vi "frameratetest.vi"() -> ()   [LabVIEW 2019]
panel:
  out "Software FPS":dbl
  out "Camera FPS":dbl
  out "Image":u16[][](graph)
  out "Camera Serial":string
  out "Camera Version":string
  out "Camera Model":string
  out "SMD":dbl
  in  "Scan Mode":dbl min=1.0 max=2.0 step=1.0
  in  "Exposure":dbl min=0.0010036691729323308 max=10.000004210526317 step=1e-08
  out "EXP":dbl
  out "SVW":i32
  out "SHW":i32
  out "SVO":i32
  out "SHO":i32
  in  "V Width":i32 min=2 max=528 step=2
  in  "V Offset":i32 min=0 max=992 step=2
  in  "H Width":i32 min=2 max=1024 step=2
  in  "H Offset":i32 min=0 max=992 step=2
  in  "Binning":u16(ring)=1 items=["1x1"=1, "2x2"=2, "4x4"=4]
  out "Elapsed Time":u32
  out "Total Frames":i32
  in  "Display":bool=TRUE
  out "error out":errorcluster
  in  "stop":bool
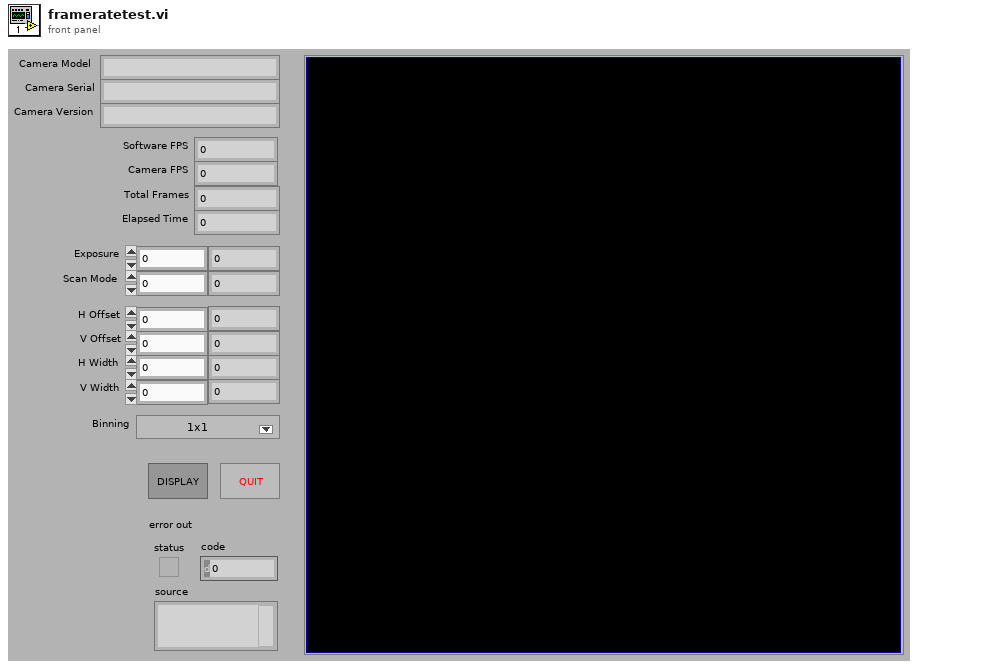
[diagram p1: front panel]
types:
  T1 = cluster{"Model":string, "Camera ID":string, "Firmware":string}
  T2 = typedef "LVMinMaxIncTypeDef.ctl" = cluster{"Minimum":dbl, "Maximum":dbl, "Increment":dbl}
  T3 = cluster{"H Offset":cluster{"Value":i32, "Limits":T2}, "V Offset":cluster{"Value":i32, "Limits":T2}, "H Size":cluster{"Value":i32, "Limits":T2}, "V Size":cluster{"Value":i32, "Limits":T2}}
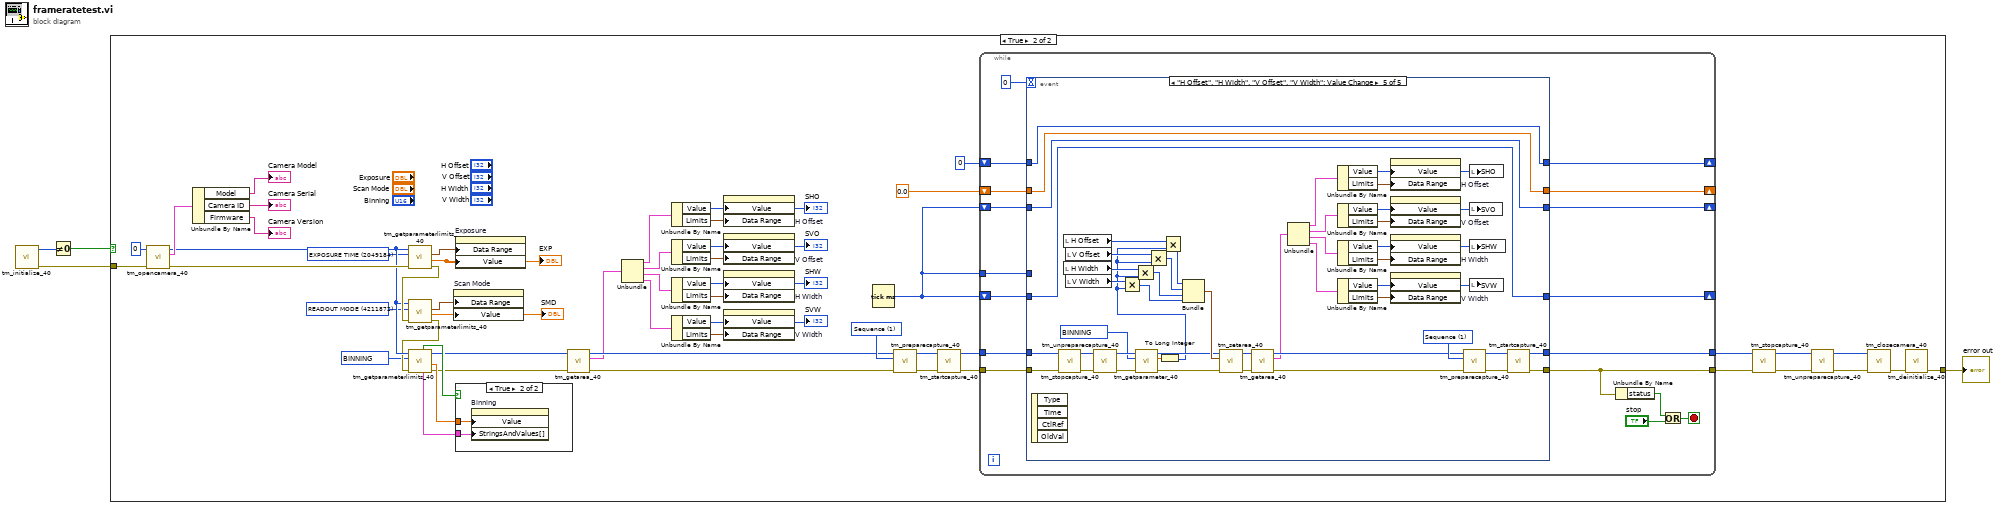
[diagram p0: block diagram]
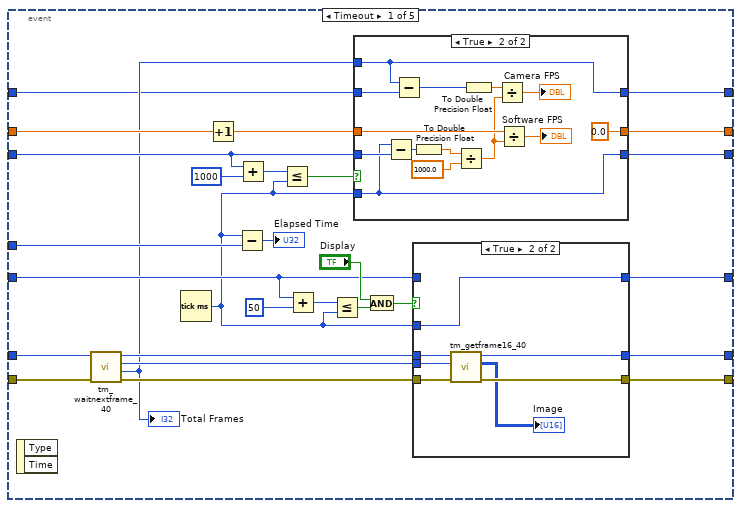
[diagram p4: hidden frame]
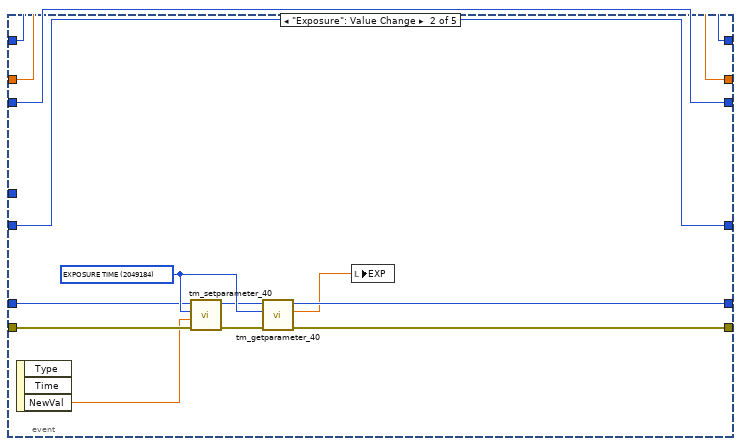
[diagram p7: hidden frame]
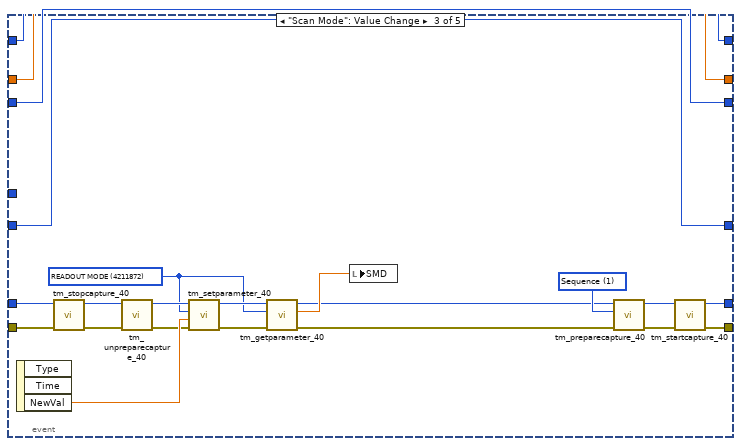
[diagram p8: hidden frame]
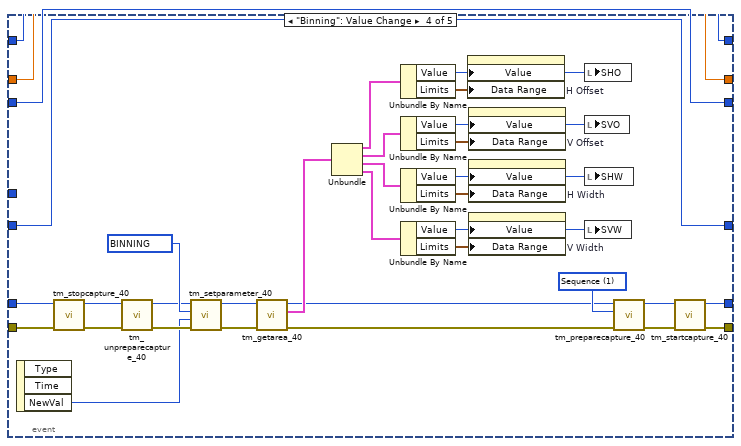
[diagram p9: hidden frame]
diagram:
  n1 = call <userlib>:"tm_initialize_40.vi"() -> ("error out"=w2:errorcluster, "Number Of Cameras"=w1:u32)  [unwired: 8 in, 2 out]
  n2 = Not Equal To 0?(x=w1) -> (x != 0?=w4:bool)
  n3 = case shown="True" w4 {
    tunnel: [w5 w55] -> w3
    tunnel: w2 -> [w5 w58]
    frame False {
    }
    frame True {
      w27 = u32 2049184 items=["BINNING"=4215968, "BITS PER CHANNEL"=4342976, "ACTIVE VIEW INDEX"=4343136, "CCD MODE"=4212384, "SENSOR MODE"=4212128, "READOUT MODE"=4211872, "EXPOSURE TIME"=2049184, "CONTRAST GAIN"=3163312, "CONTRAST OFFSET"=3163328, "LIGHT MODE"=2114720, "SENSITIVITY"=2114992, "WHITE BALANCE"=3163568, "PHOTON IMAGING MODE"=2115200, "HIGH DYNAMIC RANGE MODE"=3163360, "TRIGGER SOURCE"=1066144, "TRIGGER ACTIVE"=1066160, "TRIGGER MODE"=1066400, "TRIGGER POLARITY"=1066416, "TRIGGER GLOBAL EXPOSURE"=2049680, "FIRST TRIGGER BEHAVIOR"=2049696, "TRIGGER TIMES"=1066448, "OUTPUT TRIGGER POLARITY"=1852592, "OUTPUT TRIGGER DELAY"=1852624, "OUTPUT TRIGGER PERIOD"=1852640, "TEMPERATURE"=2115232, "TEMPERATURE TARGET"=2115264, "SENSOR COOLER FAN"=2115296, "MECHANICAL SHUTTER"=2115488, "BACK FOCUS POSITION"=8422304, "FRAMEBUNDLE MODE"=4346784, "FRAMEBUNDLE NUMBER"=4346800, "LINEBUNDLE HEIGHT"=4212192, "TRIGGER CONNECTOR"=1066432, "IMAGE PIXEL TYPE"=4343296, "OUTPUT TRIGGER KIND"=1852656, "READOUT DIRECTION"=4211904, "CHANNEL SYNC"=1852352] ("Parameter")
      w28 = u32 4211872 items=["BINNING"=4215968, "BITS PER CHANNEL"=4342976, "ACTIVE VIEW INDEX"=4343136, "CCD MODE"=4212384, "SENSOR MODE"=4212128, "READOUT MODE"=4211872, "EXPOSURE TIME"=2049184, "CONTRAST GAIN"=3163312, "CONTRAST OFFSET"=3163328, "LIGHT MODE"=2114720, "SENSITIVITY"=2114992, "WHITE BALANCE"=3163568, "PHOTON IMAGING MODE"=2115200, "HIGH DYNAMIC RANGE MODE"=3163360, "TRIGGER SOURCE"=1066144, "TRIGGER ACTIVE"=1066160, "TRIGGER MODE"=1066400, "TRIGGER POLARITY"=1066416, "TRIGGER GLOBAL EXPOSURE"=2049680, "FIRST TRIGGER BEHAVIOR"=2049696, "TRIGGER TIMES"=1066448, "OUTPUT TRIGGER POLARITY"=1852592, "OUTPUT TRIGGER DELAY"=1852624, "OUTPUT TRIGGER PERIOD"=1852640, "TEMPERATURE"=2115232, "TEMPERATURE TARGET"=2115264, "SENSOR COOLER FAN"=2115296, "MECHANICAL SHUTTER"=2115488, "BACK FOCUS POSITION"=8422304, "FRAMEBUNDLE MODE"=4346784, "FRAMEBUNDLE NUMBER"=4346800, "LINEBUNDLE HEIGHT"=4212192, "TRIGGER CONNECTOR"=1066432, "IMAGE PIXEL TYPE"=4343296, "OUTPUT TRIGGER KIND"=1852656, "READOUT DIRECTION"=4211904, "CHANNEL SYNC"=1852352] ("Parameter")
      w29 = u32 4215968 items=["BINNING"=4215968, "BITS PER CHANNEL"=4342976, "ACTIVE VIEW INDEX"=4343136, "CCD MODE"=4212384, "SENSOR MODE"=4212128, "READOUT MODE"=4211872, "EXPOSURE TIME"=2049184, "CONTRAST GAIN"=3163312, "CONTRAST OFFSET"=3163328, "LIGHT MODE"=2114720, "SENSITIVITY"=2114992, "WHITE BALANCE"=3163568, "PHOTON IMAGING MODE"=2115200, "HIGH DYNAMIC RANGE MODE"=3163360, "TRIGGER SOURCE"=1066144, "TRIGGER ACTIVE"=1066160, "TRIGGER MODE"=1066400, "TRIGGER POLARITY"=1066416, "TRIGGER GLOBAL EXPOSURE"=2049680, "FIRST TRIGGER BEHAVIOR"=2049696, "TRIGGER TIMES"=1066448, "OUTPUT TRIGGER POLARITY"=1852592, "OUTPUT TRIGGER DELAY"=1852624, "OUTPUT TRIGGER PERIOD"=1852640, "TEMPERATURE"=2115232, "TEMPERATURE TARGET"=2115264, "SENSOR COOLER FAN"=2115296, "MECHANICAL SHUTTER"=2115488, "BACK FOCUS POSITION"=8422304, "FRAMEBUNDLE MODE"=4346784, "FRAMEBUNDLE NUMBER"=4346800, "LINEBUNDLE HEIGHT"=4212192, "TRIGGER CONNECTOR"=1066432, "IMAGE PIXEL TYPE"=4343296, "OUTPUT TRIGGER KIND"=1852656, "READOUT DIRECTION"=4211904, "CHANNEL SYNC"=1852352] ("Parameter")
      w53 = 1 items=["Snap", "Sequence"] ("Capture mode")
      n4 = call <userlib>:"tm_opencamera_40.vi"("error in (no error)"=w58, "Camera Index"=u32 0) -> ("error out"=w36:errorcluster, "Camera Details"=w40:T1, "Handle out"=w34:u32)  [unwired: 7 in]
      n5 = Unbundle By Name(w40) -> ("Model"=→"Camera Model":string, "Camera ID"=→"Camera Serial":string, "Firmware"=→"Camera Version":string)
      n6 = call <userlib>:"tm_getparameterlimits_40.vi"("error in (no error)"=w36, "Parameter"=w27, "Handle in"=w34) -> ("error out"=w35:errorcluster, "default"=w19:dbl, "Range"=w20:cluster{"min":dbl, "max":dbl, "step":dbl})  [unwired: 2 in, 4 out]
      "EXP" <- w19
      n7 = call <userlib>:"tm_getparameterlimits_40.vi"("error in (no error)"=w35, "Parameter"=w28, "Handle in"=w34) -> ("error out"=w33:errorcluster, "default"=w21:dbl, "Range"=w22:cluster{"min":dbl, "max":dbl, "step":dbl})  [unwired: 2 in, 4 out]
      "SMD" <- w21
      n8 = call <userlib>:"tm_getparameterlimits_40.vi"("error in (no error)"=w33, "Parameter"=w29, "Handle in"=w34) -> ("error out"=w26:errorcluster, "default"=w31:dbl, "Handle out"=w25:u32, "Value Names"=w30:cluster{"Name":string, "Value":dbl}[], "Writable"=w32:bool)  [unwired: 2 in, 2 out]
      n9 = property on="Scan Mode" class="DigNum (strict)"("Data Range"=w22, "Value"=w21) -> ()  [unwired: 2 in, 2 out]
      n10 = property on="Exposure" class="DigNum (strict)"("Data Range"=w20, "Value"=w19) -> ()  [unwired: 2 in, 2 out]
      n11 = case shown="True" w32 {
        tunnel: w30 -> [_ w60]
        tunnel: w31 -> [_ w59]
        frame False {
        }
        frame True {
          n12 = property on="Binning" class="Ring (strict)"("Value"=w59, "StringsAndValues[]"=w60) -> ()  [unwired: 2 in, 2 out]
        }
      }
      n13 = call <userlib>:"tm_getarea_40.vi"("error in (no error)"=w26, "Handle in"=w25) -> ("error out"=w24:errorcluster, "Sub Region"=w14:T3, "Handle out"=w23:u32)  [unwired: 7 in]
      n14 = Unbundle(w14) -> ("H Offset"=w18:cluster{"Value":i32, "Limits":T2}, "V Offset"=w17:cluster{"Value":i32, "Limits":T2}, "H Size"=w16:cluster{"Value":i32, "Limits":T2}, "V Size"=w15:cluster{"Value":i32, "Limits":T2})
      n15 = Unbundle By Name(w18) -> ("Value"=w13:i32, "Limits"=w12:T2)
      "SHO" <- w13
      n16 = Unbundle By Name(w17) -> ("Value"=w7:i32, "Limits"=w6:T2)
      "SVO" <- w7
      n17 = Unbundle By Name(w16) -> ("Value"=w9:i32, "Limits"=w8:T2)
      "SHW" <- w9
      n18 = Unbundle By Name(w15) -> ("Value"=w11:i32, "Limits"=w10:T2)
      "SVW" <- w11
      n19 = property on="H Offset" class="DigNum (strict)"("Value"=w13, "Data Range"=w12) -> ()  [unwired: 2 in, 2 out]
      n20 = property on="V Offset" class="DigNum (strict)"("Value"=w7, "Data Range"=w6) -> ()  [unwired: 2 in, 2 out]
      n21 = property on="H Width" class="DigNum (strict)"("Value"=w9, "Data Range"=w8) -> ()  [unwired: 2 in, 2 out]
      n22 = property on="V Width" class="DigNum (strict)"("Value"=w11, "Data Range"=w10) -> ()  [unwired: 2 in, 2 out]
      n23 = Tick Count (ms)() -> (millisecond timer value=w48:u32)
      n24 = call <userlib>:"tm_preparecapture_40.vi"("error in (no error)"=w24, "Capture mode"=w53, "Handle in"=w23) -> ("error out"=w51:errorcluster, "Handle out"=w52:u32)  [unwired: 5 in, 2 out]
      n25 = call <userlib>:"tm_startcapture_40.vi"("error in (no error)"=w51, "Handle in"=w52) -> ("error out"=w50:errorcluster, "Handle out"=w49:u32)  [unwired: 8 in]
      n26 = while {
        tunnel: w50 -> [w67]
        tunnel: [w65] -> w47
        tunnel: [w64] -> w46
        shift-right: [w73] -> _
        shift-left: w48 -> [w71]
        shift-right: [w74] -> _
        shift-left: 0.0 -> [w72]
        shift-right: [w66] -> _
        shift-left: w48 -> [w69]
        tunnel: w49 -> [w68]
        tunnel: w48 -> [w70]
        shift-right: [w61] -> _
        shift-left: 0 -> [w62]
        stop <- w75 stop-if-true
        n27 = event shown="[4] \"H Offset\", \"H Width\", \"V Offset\", \"V Width\": Value Change" {
          selector: _ -> [_ _ _ _ _]
          dyn-events: _ -> [_ _ _ _ _]
          timeout: 0 -> [_ _ _ _ _]
          tunnel: [w82 w143 w165 w194 w240] -> w74
          tunnel: [w81 w144 w166 w195 w241] -> w73
          tunnel: w72 -> [w91 w143 w165 w194 w240]
          tunnel: w71 -> [w84 w144 w166 w195 w241]
          tunnel: w70 -> [w87 _ _ _ _]
          tunnel: w69 -> [w92 w145 w167 w201 w247]
          tunnel: w68 -> [w94 w138 w162 w193 w238]
          tunnel: w67 -> [w93 w140 w161 w192 w237]
          tunnel: [w90 w145 w167 w201 w247] -> w66
          tunnel: [w89 w135 w156 w196 w242] -> w65
          tunnel: [w88 w133 w157 w197 w243] -> w64
          tunnel: w62 -> [w79 w142 w155 w189 w234]
          tunnel: [w78 w142 w155 w189 w234] -> w61
          event Timeout {
            n28 = event-data() -> ()  [unwired: 1 in, 2 out]
            n29 = call <userlib>:"tm_waitnextframe_40.vi"("error in (no error)"=w93, "Handle in"=w94) -> ("error out"=w98:errorcluster, "Frame Count"=w80:i32, "Frame Index"=w97:i32, "Handle out"=w99:u32)  [unwired: 6 in]
            "Total Frames" <- w80
            n30 = Tick Count (ms)() -> (millisecond timer value=w86:u32)
            n31 = Increment(x=w91) -> (x+1=w83:dbl)
            n32 = Subtract(x=w86, y=w87) -> (x-y=→"Elapsed Time":u32)
            n33 = Add(x=w84, y=u32 1000) -> (x+y=w105:u32)
            n34 = Less Or Equal?(x=w105, y=w86) -> (x <= y?=w85:bool)
            n35 = Add(x=w92, y=u32 50) -> (x+y=w103:u32)
            n36 = Less Or Equal?(x=w103, y=w86) -> (x <= y?=w101:bool)
            n37 = case shown="True" w85 {
              tunnel: w84 -> [w108 w117]
              tunnel: [w108 w114] -> w81
              tunnel: w83 -> [w107 w120]
              tunnel: w86 -> [_ w114]
              tunnel: [w107 0.0] -> w82
              tunnel: w80 -> [_ w109]
              tunnel: w79 -> [w106 w112]
              tunnel: [w106 w109] -> w78
              frame False {
              }
              frame True {
                n38 = Subtract(x=w114, y=w117) -> (x-y=w116:u32)
                n39 = Subtract(x=w109, y=w112) -> (x-y=w110:i32)
                n40 = To Double Precision Float(number=w116) -> (double precision float=w122:dbl)
                n41 = Divide(x=w122, y=1000.0) -> (x/y=w113:dbl)
                n42 = To Double Precision Float(number=w110) -> (double precision float=w111:dbl)
                n43 = Divide(x=w111, y=w113) -> (x/y=→"Camera FPS":dbl)
                n44 = Divide(x=w120, y=w113) -> (x/y=→"Software FPS":dbl)
              }
            }
            n45 = And(x="Display", y=w101) -> (x .and. y?=w96:bool)
            n46 = case shown="True" w96 {
              tunnel: w92 -> [w125 _]
              tunnel: w86 -> [_ w132]
              tunnel: [w125 w132] -> w90
              tunnel: w99 -> [w124 w131]
              tunnel: w98 -> [w123 w130]
              tunnel: [w124 w129] -> w89
              tunnel: [w123 w128] -> w88
              tunnel: w97 -> [_ w126]
              frame False {
              }
              frame True {
                n47 = call <userlib>:"tm_getframe16_40.vi"("error in (no error)"=w130, "Frame Index"=w126, "Handle in"=w131) -> ("error out"=w128:errorcluster, "Data"=→"Image":u16[][], "Handle out"=w129:u32)  [unwired: 5 in, 1 out]
              }
            }
          }
          event "Exposure": Value Change {
            w141 = u32 2049184 items=["SENSOR MODE"=4212128, "CCD MODE"=4212384, "READOUT MODE"=4211872, "ACTIVE VIEW INDEX"=4343136, "BITS PER CHANNEL"=4342976, "IMAGE PIXEL TYPE"=4343296, "BINNING"=4215968, "EXPOSURE TIME"=2049184, "CONTRAST GAIN"=3163312, "CONTRAST OFFSET"=3163328, "LIGHT MODE"=2114720, "SENSITIVITY"=2114992, "PHOTON IMAGING MODE"=2115200, "HIGH DYNAMIC RANGE MODE"=3163360, "WHITE BALANCE"=3163568, "TEMPERATURE"=2115232, "TEMPERATURE TARGET"=2115264, "SENSOR COOLER FAN"=2115296, "LINEBUNDLE HEIGHT"=4212192, "MECHANICAL SHUTTER"=2115488, "BACK FOCUS POSITION"=8422304, "TRIGGER CONNECTOR"=1066432, "TRIGGER SOURCE"=1066144, "OUTPUT TRIGGER SOURCE"=1852576, "TRIGGER GLOBAL EXPOSURE"=2049680, "FIRST TRIGGER BEHAVIOR"=2049696, "CHANNEL SYNC"=1852352, "READOUT DIRECTION"=4211904, "PRE HSYNC COUNT"=1852704] ("Parameter")
            n48 = event-data() -> ("NewVal"=w139:dbl)  [unwired: 1 in, 2 out]
            n49 = call <userlib>:"tm_setparameter_40.vi"("error in (no error)"=w140, "Value in"=w139, "Parameter"=w141, "Handle in"=w138) -> ("error out"=w137:errorcluster, "Handle out"=w136:u32)  [unwired: 6 in]
            n50 = call <userlib>:"tm_getparameter_40.vi"("error in (no error)"=w137, "Parameter"=w141, "Handle in"=w136) -> ("error out"=w133:errorcluster, "Value out"=w134:dbl, "Handle out"=w135:u32)  [unwired: 6 in]
            n51 = local write "EXP"(w134) -> ()
          }
          event "Scan Mode": Value Change {
            w146 = u32 4211872 items=["SENSOR MODE"=4212128, "CCD MODE"=4212384, "READOUT MODE"=4211872, "ACTIVE VIEW INDEX"=4343136, "BITS PER CHANNEL"=4342976, "IMAGE PIXEL TYPE"=4343296, "BINNING"=4215968, "EXPOSURE TIME"=2049184, "CONTRAST GAIN"=3163312, "CONTRAST OFFSET"=3163328, "LIGHT MODE"=2114720, "SENSITIVITY"=2114992, "PHOTON IMAGING MODE"=2115200, "HIGH DYNAMIC RANGE MODE"=3163360, "WHITE BALANCE"=3163568, "TEMPERATURE"=2115232, "TEMPERATURE TARGET"=2115264, "SENSOR COOLER FAN"=2115296, "LINEBUNDLE HEIGHT"=4212192, "MECHANICAL SHUTTER"=2115488, "BACK FOCUS POSITION"=8422304, "TRIGGER CONNECTOR"=1066432, "TRIGGER SOURCE"=1066144, "OUTPUT TRIGGER SOURCE"=1852576, "TRIGGER GLOBAL EXPOSURE"=2049680, "FIRST TRIGGER BEHAVIOR"=2049696, "CHANNEL SYNC"=1852352, "READOUT DIRECTION"=4211904, "PRE HSYNC COUNT"=1852704] ("Parameter")
            w160 = 1 items=["Snap", "Sequence"] ("Capture mode")
            n52 = event-data() -> ("NewVal"=w151:dbl)  [unwired: 1 in, 2 out]
            n53 = call <userlib>:"tm_stopcapture_40.vi"("error in (no error)"=w161, "Handle in"=w162) -> ("error out"=w163:errorcluster, "Handle out"=w164:u32)  [unwired: 8 in]
            n54 = call <userlib>:"tm_unpreparecapture_40.vi"("error in (no error)"=w163, "Handle in"=w164) -> ("error out"=w149:errorcluster, "Handle out"=w150:u32)  [unwired: 8 in]
            n55 = call <userlib>:"tm_setparameter_40.vi"("error in (no error)"=w149, "Value in"=w151, "Parameter"=w146, "Handle in"=w150) -> ("error out"=w148:errorcluster, "Handle out"=w147:u32)  [unwired: 6 in]
            n56 = call <userlib>:"tm_getparameter_40.vi"("error in (no error)"=w148, "Parameter"=w146, "Handle in"=w147) -> ("error out"=w154:errorcluster, "Value out"=w153:dbl, "Handle out"=w152:u32)  [unwired: 6 in]
            n57 = local write "SMD"(w153) -> ()
            n58 = call <userlib>:"tm_preparecapture_40.vi"("error in (no error)"=w154, "Capture mode"=w160, "Handle in"=w152) -> ("error out"=w158:errorcluster, "Handle out"=w159:u32)  [unwired: 5 in, 2 out]
            n59 = call <userlib>:"tm_startcapture_40.vi"("error in (no error)"=w158, "Handle in"=w159) -> ("error out"=w157:errorcluster, "Handle out"=w156:u32)  [unwired: 8 in]
          }
          event "Binning": Value Change {
            w187 = u32 4215968 items=["BINNING"=4215968, "BITS PER CHANNEL"=2, "ACTIVE VIEW INDEX"=3, "CCD MODE"=4, "SENSOR MODE"=5, "READOUT MODE"=6, "EXPOSURE TIME"=7, "CONTRAST GAIN"=8, "CONTRAST OFFSET"=9, "LIGHT MODE"=10, "SENSITIVITY"=11, "WHITE BALANCE"=12, "PHOTON IMAGING MODE"=13, "HIGH DYNAMIC RANGE MODE"=14, "TRIGGER SOURCE"=15, "TRIGGER ACTIVE"=16, "TRIGGER MODE"=17, "TRIGGER POLARITY"=18, "TRIGGER GLOBAL EXPOSURE"=19, "FIRST TRIGGER BEHAVIOR"=20, "TRIGGER TIMES"=21, "OUTPUT TRIGGER POLARITY"=22, "OUTPUT TRIGGER DELAY"=23, "OUTPUT TRIGGER PERIOD"=24, "TEMPERATURE"=25, "TEMPERATURE TARGET"=26, "SENSOR COOLER FAN"=27, "MECHANICAL SHUTTER"=28, "BACK FOCUS POSITION"=29, "FRAMEBUNDLE MODE"=30, "FRAMEBUNDLE NUMBER"=31, "LINEBUNDLE HEIGHT"=32, "TRIGGER CONNECTOR"=33, "IMAGE PIXEL TYPE"=34, "OUTPUT TRIGGER KIND"=35, "READOUT DIRECTION"=36, "CHANNEL SYNC"=37] ("Parameter")
            w200 = 1 items=["Snap", "Sequence"] ("Capture mode")
            n60 = event-data() -> ("NewVal"=w185:u16)  [unwired: 1 in, 2 out]
            n61 = call <userlib>:"tm_stopcapture_40.vi"("error in (no error)"=w192, "Handle in"=w193) -> ("error out"=w190:errorcluster, "Handle out"=w191:u32)  [unwired: 8 in]
            n62 = call <userlib>:"tm_unpreparecapture_40.vi"("error in (no error)"=w190, "Handle in"=w191) -> ("error out"=w188:errorcluster, "Handle out"=w186:u32)  [unwired: 8 in]
            n63 = call <userlib>:"tm_setparameter_40.vi"("error in (no error)"=w188, "Value in"=w185, "Parameter"=w187, "Handle in"=w186) -> ("error out"=w182:errorcluster, "Handle out"=w183:u32)  [unwired: 6 in]
            n64 = call <userlib>:"tm_getarea_40.vi"("error in (no error)"=w182, "Handle in"=w183) -> ("error out"=w180:errorcluster, "Sub Region"=w184:T3, "Handle out"=w181:u32)  [unwired: 7 in]
            n65 = Unbundle(w184) -> ("H Offset"=w171:cluster{"Value":i32, "Limits":T2}, "V Offset"=w170:cluster{"Value":i32, "Limits":T2}, "H Size"=w169:cluster{"Value":i32, "Limits":T2}, "V Size"=w168:cluster{"Value":i32, "Limits":T2})
            n66 = Unbundle By Name(w171) -> ("Value"=w179:i32, "Limits"=w178:T2)
            n67 = Unbundle By Name(w170) -> ("Value"=w177:i32, "Limits"=w176:T2)
            n68 = Unbundle By Name(w169) -> ("Value"=w175:i32, "Limits"=w174:T2)
            n69 = Unbundle By Name(w168) -> ("Value"=w173:i32, "Limits"=w172:T2)
            n70 = property on="H Offset" class="DigNum (strict)"("Value"=w179, "Data Range"=w178) -> ()  [unwired: 2 in, 2 out]
            n71 = property on="V Offset" class="DigNum (strict)"("Value"=w177, "Data Range"=w176) -> ()  [unwired: 2 in, 2 out]
            n72 = property on="H Width" class="DigNum (strict)"("Value"=w175, "Data Range"=w174) -> ()  [unwired: 2 in, 2 out]
            n73 = property on="V Width" class="DigNum (strict)"("Value"=w173, "Data Range"=w172) -> ()  [unwired: 2 in, 2 out]
            n74 = local write "SHO"(w179) -> ()
            n75 = local write "SVO"(w177) -> ()
            n76 = local write "SHW"(w175) -> ()
            n77 = local write "SVW"(w173) -> ()
            n78 = call <userlib>:"tm_preparecapture_40.vi"("error in (no error)"=w180, "Capture mode"=w200, "Handle in"=w181) -> ("error out"=w198:errorcluster, "Handle out"=w199:u32)  [unwired: 5 in, 2 out]
            n79 = call <userlib>:"tm_startcapture_40.vi"("error in (no error)"=w198, "Handle in"=w199) -> ("error out"=w197:errorcluster, "Handle out"=w196:u32)  [unwired: 8 in]
          }
          event "H Offset", "H Width", "V Offset", "V Width": Value Change {
            w214 = u32 4215968 items=["SENSOR MODE"=4212128, "READOUT SPEED"=4211872, "READOUT DIRECTION"=4211904, "TRIGGER GLOBAL EXPOSURE"=2049680, "TRIGGER DELAY"=1066480, "INTERNAL TRIGGER HANDLING"=1066496, "SENSOR TEMPERATURE"=2115232, "SENSOR COOLER STATUS"=2115280, "EXPOSURE TIME"=2049184, "DEFECT CORRECT MODE"=4670368, "HOT PIXEL CORRECT LEVEL"=4670400, "BINNING"=4215968, "TIMING READOUT TIME"=4223904, "INTERNAL FRAME RATE"=4225952, "INTERNAL FRAME INTERVAL"=4225968, "INTERNAL LINE SPEED"=4226000, "INTERNAL LINE INTERVAL"=4226016, "IMAGE WIDTH"=4343200, "IMAGE HEIGHT"=4343216, "IMAGE ROWBYTES"=4343232, "IMAGE FRAMEBYTES"=4343248, "IMAGE PIXEL TYPE"=4343296, "NUMBER OF OUTPUT TRIGGER CONNECTOR"=1852320, "OUTPUT TRIGGER SOURCE[0]"=1852576, "OUTPUT TRIGGER SOURCE[1]"=1852832, "OUTPUT TRIGGER SOURCE[2]"=1853088, "OUTPUT TRIGGER POLARITY[0]"=1852592, "OUTPUT TRIGGER POLARITY[1]"=1852848, "OUTPUT TRIGGER POLARITY[2]"=1853104, "OUTPUT TRIGGER ACTIVE[0]"=1852608, "OUTPUT TRIGGER ACTIVE[1]"=1852864, "OUTPUT TRIGGER ACTIVE[2]"=1853120, "OUTPUT TRIGGER DELAY[0]"=1852624, "OUTPUT TRIGGER DELAY[1]"=1852880, "OUTPUT TRIGGER DELAY[2]"=1853136, "OUTPUT TRIGGER PERIOD[0]"=1852640, "OUTPUT TRIGGER PERIOD[1]"=1852896, "OUTPUT TRIGGER PERIOD[2]"=1853152, "OUTPUT TRIGGER KIND[0]"=1852656, "OUTPUT TRIGGER KIND[1]"=1852912, "OUTPUT TRIGGER KIND[2]"=1853168, "OUTPUT TRIGGER BASE SENSOR[0]"=1852672, "OUTPUT TRIGGER BASE SENSOR[1]"=1852928, "OUTPUT TRIGGER BASE SENSOR[2]"=1853184, "OUTPUT TRIGGER PRE HSYNC COUNT"=1852704] ("Parameter")
            w246 = 1 items=["Snap", "Sequence"] ("Capture mode")
            n80 = event-data() -> ()  [unwired: 1 in, 4 out]
            n81 = call <userlib>:"tm_stopcapture_40.vi"("error in (no error)"=w237, "Handle in"=w238) -> ("error out"=w235:errorcluster, "Handle out"=w236:u32)  [unwired: 8 in]
            n82 = local read "H Offset"() -> (w211:i32)
            n83 = local read "H Width"() -> (w209:i32)
            n84 = local read "V Offset"() -> (w210:i32)
            n85 = local read "V Width"() -> (w208:i32)
            n86 = call <userlib>:"tm_unpreparecapture_40.vi"("error in (no error)"=w235, "Handle in"=w236) -> ("error out"=w215:errorcluster, "Handle out"=w216:u32)  [unwired: 8 in]
            n87 = call <userlib>:"tm_getparameter_40.vi"("error in (no error)"=w215, "Parameter"=w214, "Handle in"=w216) -> ("error out"=w212:errorcluster, "Value out"=w203:dbl, "Handle out"=w213:u32)  [unwired: 6 in]
            n88 = To Long Integer(number=w203) -> (32bit integer=w202:i32)
            n89 = Multiply(x=w208, y=w202) -> (x*y=w204:i32)
            n90 = Multiply(x=w209, y=w202) -> (x*y=w205:i32)
            n91 = Multiply(x=w210, y=w202) -> (x*y=w206:i32)
            n92 = Multiply(x=w211, y=w202) -> (x*y=w207:i32)
            n93 = Bundle(w207, w206, w205, w204) -> (w239:cluster{i32, i32, i32, i32})  [unwired: 1 in]
            n94 = call <userlib>:"tm_setarea_40.vi"("error in (no error)"=w212, "Sub Region"=w239, "Handle in"=w213) -> ("error out"=w232:errorcluster, "Handle out"=w233:u32)  [unwired: 7 in]
            n95 = call <userlib>:"tm_getarea_40.vi"("error in (no error)"=w232, "Handle in"=w233) -> ("error out"=w230:errorcluster, "Sub Region"=w222:T3, "Handle out"=w231:u32)  [unwired: 7 in]
            n96 = Unbundle(w222) -> ("H Offset"=w229:cluster{"Value":i32, "Limits":T2}, "V Offset"=w228:cluster{"Value":i32, "Limits":T2}, "H Size"=w227:cluster{"Value":i32, "Limits":T2}, "V Size"=w226:cluster{"Value":i32, "Limits":T2})
            n97 = Unbundle By Name(w229) -> ("Value"=w225:i32, "Limits"=w224:T2)
            n98 = Unbundle By Name(w228) -> ("Value"=w223:i32, "Limits"=w218:T2)
            n99 = Unbundle By Name(w227) -> ("Value"=w219:i32, "Limits"=w217:T2)
            n100 = Unbundle By Name(w226) -> ("Value"=w221:i32, "Limits"=w220:T2)
            n101 = property on="H Offset" class="DigNum (strict)"("Value"=w225, "Data Range"=w224) -> ()  [unwired: 2 in, 2 out]
            n102 = property on="V Offset" class="DigNum (strict)"("Value"=w223, "Data Range"=w218) -> ()  [unwired: 2 in, 2 out]
            n103 = property on="H Width" class="DigNum (strict)"("Value"=w219, "Data Range"=w217) -> ()  [unwired: 2 in, 2 out]
            n104 = property on="V Width" class="DigNum (strict)"("Value"=w221, "Data Range"=w220) -> ()  [unwired: 2 in, 2 out]
            n105 = call <userlib>:"tm_preparecapture_40.vi"("error in (no error)"=w230, "Capture mode"=w246, "Handle in"=w231) -> ("error out"=w244:errorcluster, "Handle out"=w245:u32)  [unwired: 5 in, 2 out]
            n106 = local write "SHO"(w225) -> ()
            n107 = local write "SVO"(w223) -> ()
            n108 = local write "SHW"(w219) -> ()
            n109 = local write "SVW"(w221) -> ()
            n110 = call <userlib>:"tm_startcapture_40.vi"("error in (no error)"=w244, "Handle in"=w245) -> ("error out"=w243:errorcluster, "Handle out"=w242:u32)  [unwired: 8 in]
          }
        }
        n111 = Unbundle By Name(w64) -> ("status"=w76:bool)
        n112 = Or(x=w76, y="stop") -> (x .or. y?=w75:bool)
      }
      n113 = call <userlib>:"tm_stopcapture_40.vi"("error in (no error)"=w46, "Handle in"=w47) -> ("error out"=w43:errorcluster, "Handle out"=w44:u32)  [unwired: 8 in]
      n114 = call <userlib>:"tm_unpreparecapture_40.vi"("error in (no error)"=w43, "Handle in"=w44) -> ("error out"=w42:errorcluster, "Handle out"=w45:u32)  [unwired: 8 in]
      n115 = call <userlib>:"tm_closecamera_40.vi"("error in (no error)"=w42, "Handle in"=w45) -> ("error out"=w56:errorcluster)  [unwired: 9 in]
      n116 = call <userlib>:"tm_deinitialize_40.vi"("error in (no error)"=w56) -> ("error out"=w55:errorcluster)  [unwired: 10 in]
    }
  }
  "error out" <- w3
